vi "RichToFlatni_measurementlink_discovery_v1_EnumerateServicesResponse.vi"(5 "OutputClusterType":T1, 11 "InputCluster":T4) -> (3 "OutputCluster":T1)   [LabVIEW 2021, in "ni.measurementlink.discovery.v1.api.lvlib"]
uses:
  ni_measurementlink_discovery_v1_EnumerateServicesResponse.ctl
  ni_measurementlink_discovery_v1_ServiceDescriptor.ctl
  ni_measurementlink_discovery_v1_ServiceDescriptor_AnnotationsEntry.ctl
  ni_measurementlink_discovery_v1_EnumerateServicesResponse_Flat.ctl
  ni_measurementlink_discovery_v1_ServiceDescriptor_Flat.ctl
  ni_measurementlink_discovery_v1_ServiceDescriptor_AnnotationsEntry_Flat.ctl
  ni.measurementlink.discovery.v1.api.lvlib
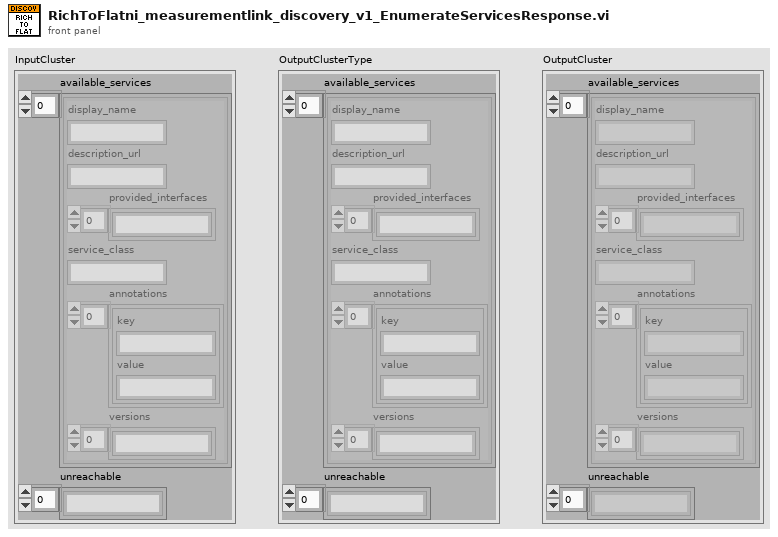
[diagram p1: front panel]
types:
  T1 = typedef "ni.measurementlink.discovery.v1.api.lvlib/ni_measurementlink_discovery_v1_EnumerateServicesResponse_Flat.ctl" = cluster{"available_services":T2[], "unreachable":string[]}
  T2 = typedef "ni.measurementlink.discovery.v1.api.lvlib/ni_measurementlink_discovery_v1_ServiceDescriptor_Flat.ctl" = cluster{"display_name":string, "description_url":string, "provided_interfaces":string[], "service_class":string, "annotations":T3[], "versions":string[]}
  T3 = typedef "ni.measurementlink.discovery.v1.api.lvlib/ni_measurementlink_discovery_v1_ServiceDescriptor_AnnotationsEntry_Flat.ctl" = cluster{"key":string, "value":string}
  T4 = typedef "ni.measurementlink.discovery.v1.api.lvlib/ni_measurementlink_discovery_v1_EnumerateServicesResponse.ctl" = cluster{"available_services":T5[], "unreachable":string[]}
  T5 = typedef "ni.measurementlink.discovery.v1.api.lvlib/ni_measurementlink_discovery_v1_ServiceDescriptor.ctl" = cluster{"display_name":string, "description_url":string, "provided_interfaces":string[], "service_class":string, "annotations":T6[], "versions":string[]}
  T6 = typedef "ni.measurementlink.discovery.v1.api.lvlib/ni_measurementlink_discovery_v1_ServiceDescriptor_AnnotationsEntry.ctl" = cluster{"key":string, "value":string}
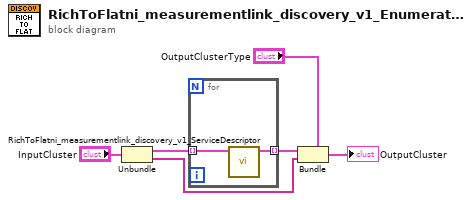
[diagram p0: block diagram]
diagram:
  n1 = Unbundle "Unbundle"("InputCluster") -> ("available_services"=w3:T5[], "unreachable"=w1:string[])
  n2 = for {
    tunnel: w3 -> [w8] mode=indexing
    tunnel: [w7] -> w2 mode=indexing
    n3 = call "RichToFlatni_measurementlink_discovery_v1_ServiceDescriptor.vi"("InputCluster"=w8) -> ("OutputCluster"=w7:T2)  [unwired: 10 in]
  }
  n4 = Bundle "Bundle"(cluster="OutputClusterType", "available_services"=w2, "unreachable"=w1) -> (→"OutputCluster":T1)
